vi "Insert Space in Korean.vi"(8 "error in (no error)":errorcluster caption="에러 입력(에러 없음)", 10 "in":string) -> (0 "error out":errorcluster caption="에러 출력", 2 "out":string)   [LabVIEW 2020]
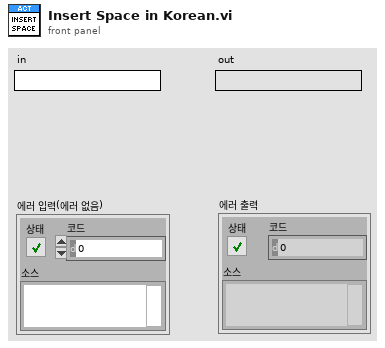
[diagram p1: front panel]
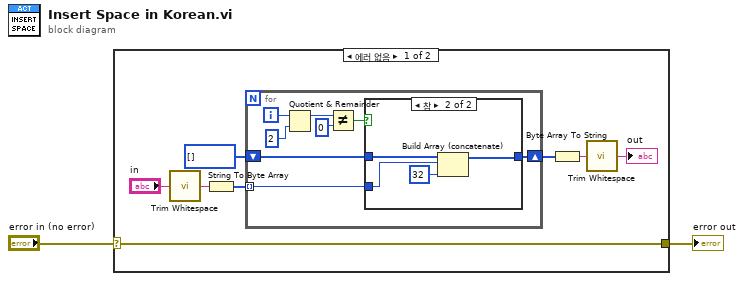
[diagram p0: block diagram]
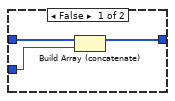
[diagram p2: hidden frame]
diagram:
  n1 = case shown="에러 없음" "error in (no error)" {
    selector: "error in (no error)" -> [w5 w26]
    tunnel: [w5 w26] -> w1
    frame No Error {
      n2 = call <vilib>:"Trim Whitespace.vi"("string"="in") -> ("trimmed string"=w4:string)  [unwired: 1 in]
      n3 = String To Byte Array(string=w4) -> (unsigned byte array=w10:u8[])
      n4 = for {
        tunnel: w10 -> [w13] mode=indexing
        shift-right: [w12] -> w8
        shift-left: u8[] [] -> [w11]
        i -> [w18]
        n5 = Quotient & Remainder(x=w18, y=2) -> (x-y*floor(x/y)=w16:i32)  [unwired: 1 out]
        n6 = Not Equal?(x=w16, y=0) -> (x != y?=w14:bool)
        n7 = case shown="참" w14 {
          tunnel: w13 -> [w19 w25]
          tunnel: [w20 w24] -> w12
          tunnel: w11 -> [w21 w23]
          frame False {
            n8 = Build Array (concatenate)(w21, w19) -> (w20:u8[])
          }
          frame True {
            n9 = Build Array (concatenate)(w23, w25, u8 32) -> (w24:u8[])
          }
        }
      }
      n10 = Byte Array To String(unsigned byte array=w8) -> (string=w6:string)
      n11 = call <vilib>:"Trim Whitespace.vi"("string"=w6) -> ("trimmed string"=→"out":string)  [unwired: 1 in]
    }
    frame Error {
    }
  }
  "error out" <- w1
